vi "Read Max Voltage.vi"(11 "E3610x in":refnum<class "E3610x.lvclass">) -> (2 "Max Voltage":dbl, 3 "E3610x out":refnum<class "E3610x.lvclass">)   [LabVIEW 2020, in "E3610x.lvclass"]
uses:
  E3610x.lvclass
  E3610x.lvclass/E3610x.ctl
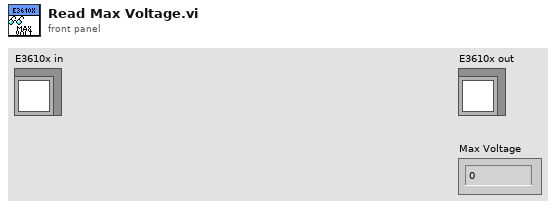
[diagram p1: front panel]
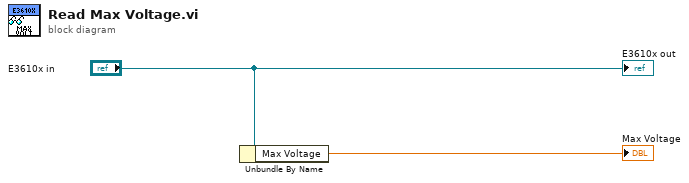
[diagram p0: block diagram]
diagram:
  n1 = Unbundle By Name("E3610x in") -> ("Max Voltage"=→"Max Voltage":dbl)
  "E3610x out" <- "E3610x in"
